vi "Move Joints.vi"(4 "Side":T1, 5 "Label":string, 6 "Wait (s)":dbl, 8 "error in":errorcluster, 9 "time":dbl=2.0, 10 "Goal":dbl[](array[numeric])) -> (0 "error out":errorcluster, 2 "Goal":dbl[](array[numeric]))   [LabVIEW 2013]
uses:
  ROS/Code/SubVIs/BaxterSide.ctl
  ROS/Code/Console/Servers/ServerSubs/(nist) Arm Globals.vi
panel:
  # "All Joint motions\nare relative to BASE"
  # "Cannot make\njoint motions \nvertical"
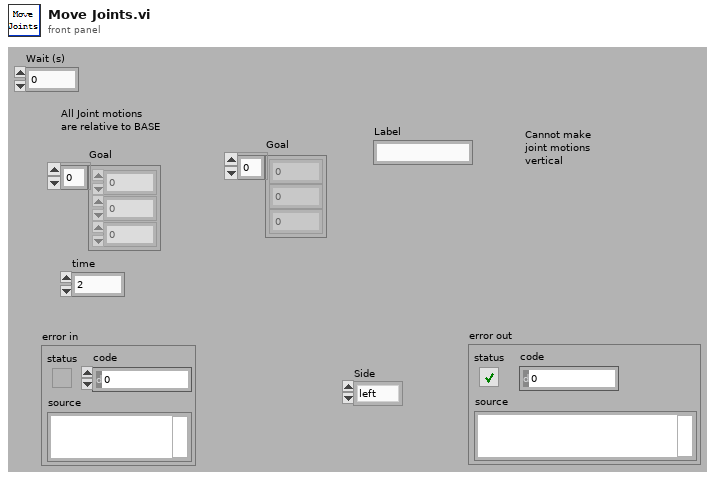
[diagram p1: front panel]
types:
  T1 = typedef "BaxterSide.ctl" = enum16{"left", "right"}
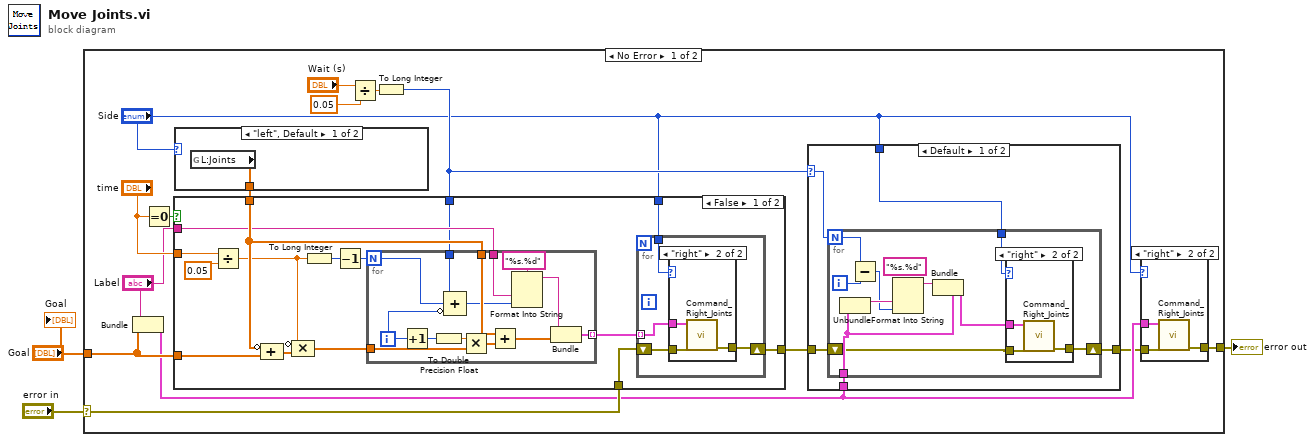
[diagram p0: block diagram]
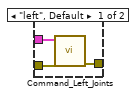
[diagram p2: hidden frame]
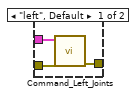
[diagram p3: hidden frame]
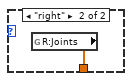
[diagram p5: hidden frame]
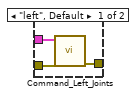
[diagram p6: hidden frame]
diagram:
  n1 = case shown="No Error" "error in" {
    selector: "error in" -> [w8 w89]
    tunnel: [w7 w89] -> w2
    tunnel: "Goal" -> [w9 _]
    frame No Error {
      n2 = Bundle("Label"="Label", "Goal"=w9) -> (w6:cluster{"Label":string, "Goal":dbl[]})  [unwired: 1 in]
      n3 = Equal To 0?(x="time") -> (x = 0?=w18:bool)
      n4 = case shown="\"left\", Default" "Side" {
        tunnel: [w47 w48] -> w17
        frame "left", Default {
          n5 = global read "(nist) Arm Globals.vi" "L:Joints"() -> (w47:dbl[])
        }
        frame "right" {
          n6 = global read "(nist) Arm Globals.vi" "R:Joints"() -> (w48:dbl[])
        }
      }
      n7 = Divide(x="Wait (s)", y=0.05) -> (x/y=w12:dbl)
      n8 = To Long Integer(number=w12) -> (32bit integer=w11:i32)
      n9 = case shown="False" w18 {
        tunnel: "Label" -> [w58 _]
        tunnel: w9 -> [w61 _]
        tunnel: w17 -> [w59 _]
        tunnel: "time" -> [w63 _]
        tunnel: w11 -> [w53 _]
        tunnel: [w51 w88] -> w10
        tunnel: "Side" -> [w50 _]
        tunnel: w8 -> [w49 w88]
        frame False {
          n10 = Divide(x=w63, y=0.05) -> (x/y=w54:dbl)
          n11 = Compound Arithmetic op=ADD(invert w59, w61) -> (w55:dbl[])
          n12 = Compound Arithmetic op=MULTIPLY(invert w54, w55) -> (w56:dbl[])
          n13 = To Long Integer(number=w54) -> (32bit integer=w60:i32)
          n14 = Decrement(x=w60) -> (x-1=w57:i32)
          n15 = for {
            N: w57 -> [w83]
            tunnel: w59 -> [w87]
            tunnel: w56 -> [w80]
            tunnel: w58 -> [w78]
            tunnel: [w84] -> w52 mode=indexing
            tunnel: w53 -> [w74]
            i -> [w82]
            n16 = Increment(x=w82) -> (x+1=w75:i32)
            n17 = To Double Precision Float(number=w75) -> (double precision float=w81:dbl)
            n18 = Compound Arithmetic op=ADD(w74, w83, invert w82) -> (w77:i32)
            n19 = Multiply(x=w81, y=w80) -> (x*y=w86:dbl[])
            n20 = Add(x=w87, y=w86) -> (x+y=w85:dbl[])
            n21 = Format Into String(format string="%s.%d", w78, w77) -> (resulting string=w76:string)  [unwired: 2 in, 1 out]
            n22 = Bundle(w76, w85) -> (w84:cluster{string, dbl[]})  [unwired: 1 in]
          }
          n23 = for {
            tunnel: w52 -> [w66] mode=indexing
            shift-right: [w64] -> w51
            shift-left: w49 -> [w65]
            tunnel: w50 -> [w67]
            n24 = case shown="\"right\"" w67 {
              tunnel: w66 -> [w70 w73]
              tunnel: w65 -> [w69 w72]
              tunnel: [w68 w71] -> w64
              frame "left", Default {
                n25 = call "Command_Left_Joints.vi"("error in"=w69, "Goal"=w70) -> ("error out"=w68:errorcluster)  [unwired: 6 in, 1 out]
              }
              frame "right" {
                n26 = call "Command_Right_Joints.vi"("error in"=w72, "Goal"=w73) -> ("error out"=w71:errorcluster)  [unwired: 6 in, 1 out]
              }
            }
          }
        }
        frame True {
        }
      }
      n27 = case shown="Default" w11 {
        selector: w11 -> [w26 _]
        tunnel: w10 -> [w29 w46]
        tunnel: [w28 w46] -> w5
        tunnel: w6 -> [w27 _]
        tunnel: "Side" -> [w25 _]
        frame Default {
          n28 = for {
            N: w26 -> [w39]
            tunnel: w27 -> [w34]
            shift-right: [w33] -> w28
            shift-left: w29 -> [w32]
            tunnel: w25 -> [w30]
            i -> [w38]
            (unwired) "%s.%d" ("format string")
            n29 = Unbundle(w34) -> ("Label"=w37:string)  [unwired: 1 out]
            n30 = Subtract(x=w39, y=w38) -> (x-y=w36:i32)
            n31 = Format Into String(w37, w36) -> (resulting string=w35:string)  [unwired: 3 in, 1 out]
            n32 = Bundle(cluster=w34, "Label"=w35) -> (w31:cluster{"Label":string, "Goal":dbl[]})  [unwired: 1 in]
            n33 = case shown="\"right\"" w30 {
              tunnel: w31 -> [w42 w45]
              tunnel: w32 -> [w41 w44]
              tunnel: [w40 w43] -> w33
              frame "left", Default {
                n34 = call "Command_Left_Joints.vi"("error in"=w41, "Goal"=w42) -> ("error out"=w40:errorcluster)  [unwired: 6 in, 1 out]
              }
              frame "right" {
                n35 = call "Command_Right_Joints.vi"("error in"=w44, "Goal"=w45) -> ("error out"=w43:errorcluster)  [unwired: 6 in, 1 out]
              }
            }
          }
        }
        frame 0 {
        }
      }
      n36 = case shown="\"right\"" "Side" {
        tunnel: w6 -> [w21 w24]
        tunnel: w5 -> [w20 w23]
        tunnel: [w19 w22] -> w7
        frame "left", Default {
          n37 = call "Command_Left_Joints.vi"("error in"=w20, "Goal"=w21) -> ("error out"=w19:errorcluster)  [unwired: 6 in, 1 out]
        }
        frame "right" {
          n38 = call "Command_Right_Joints.vi"("error in"=w23, "Goal"=w24) -> ("error out"=w22:errorcluster)  [unwired: 6 in, 1 out]
        }
      }
    }
    frame Error {
    }
  }
  "error out" <- w2
  "Goal" <- "Goal"
